vi "AVG Irms.vi"(9 "Line 3":waveform(dbl), 10 "Line 2":waveform(dbl), 11 "Line 1":waveform(dbl)) -> (3 "AVG RMS":dbl)   [LabVIEW 2019]
uses:
  <vilib>/measure/madcrms.llb/Basic Averaged DC-RMS for 1 Chan.vi
  <vilib>/measure/NI_MAPro.lvlib
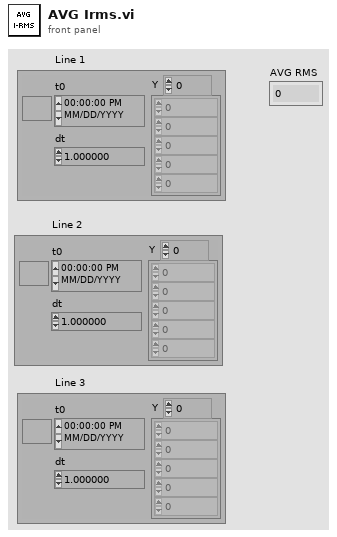
[diagram p1: front panel]
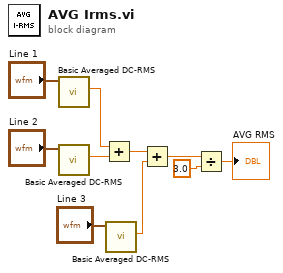
[diagram p0: block diagram]
diagram:
  n1 = call-poly <vilib>:"Basic Averaged DC-RMS.vi"("signal in"="Line 1") -> ("RMS value"=w10:dbl)  [unwired: 7 in, 3 out]
  n2 = call-poly <vilib>:"Basic Averaged DC-RMS.vi"("signal in"="Line 2") -> ("RMS value"=w9:dbl)  [unwired: 7 in, 3 out]
  n3 = Add(x=w10, y=w9) -> (x+y=w8:dbl)
  n4 = call-poly <vilib>:"Basic Averaged DC-RMS.vi"("signal in"="Line 3") -> ("RMS value"=w7:dbl)  [unwired: 7 in, 3 out]
  n5 = Add(x=w8, y=w7) -> (x+y=w6:dbl)
  n6 = Divide(x=w6, y=3.0) -> (x/y=→"AVG RMS":dbl)
